vi "3D-SplitterROIClusterToString.vi"(0 "Rectangle":T1 {"Rotation" format="%.2f"; "Left" scale=0.0..1024.0; "Right" scale=0.0..1024.0}) -> (14 "Roi":string[](array[string]))   [LabVIEW 2015]
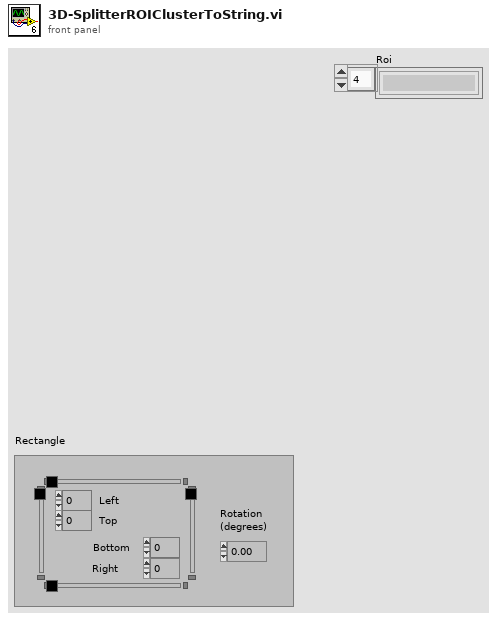
[diagram p1: front panel]
types:
  T1 = typedef "IMAQ Rectangle" = cluster{"Left":i32, "Top":i32, "Right":i32, "Bottom":i32, "Rotation":dbl}
  T2 = cluster{"Left":string, "Top":string, "Right":string, "Bottom":string, "Rotation":string}
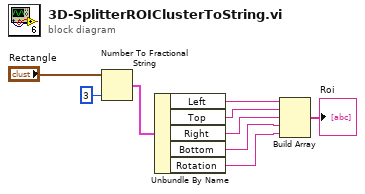
[diagram p0: block diagram]
diagram:
  n1 = Number To Fractional String(number="Rectangle", precision (6)=i16 3 ("精度(6)")) -> (F-format string=w7:T2)  [unwired: 2 in]
  n2 = Unbundle By Name(w7) -> ("Left"=w6:string, "Top"=w5:string, "Right"=w4:string, "Bottom"=w3:string, "Rotation"=w2:string)
  n3 = Build Array(w6, w5, w4, w3, w2) -> (→"Roi":string[])
